vi "GPS Trail.vi"() -> ()   [LabVIEW 2009]
uses:
  <vilib>/Platform/TimedLoop/XDataNode/XDataNode.xnode
  <vilib>/Platform/TimedLoop/XDataNode/nitl_modes.ctl
  <vilib>/Platform/TimedLoop/XDataNode/XDNodeRunTimeDep.lvlib
  <vilib>/Platform/TimedLoop/XDataNode/wakeup.ctl
  <vilib>/Platform/TimedLoop/XDataNode/timing_clust.ctl
  <vilib>/Platform/TimedLoop/XDataNode/loadlvalarms.vi
  <vilib>/Analysis/NI_AALBase.lvlib
  TypeDefs/Sensor TypeDefs/GPS Data.ctl
  Functional Global Variables/Actions for FG's.ctl
panel:
  out "Latitude point sample":dbl format="%0.2f"
  out "Longitude point sample":dbl format="%0.2f"
  out "Latitude Array":dbl[](array[numeric]) format="%#_12g"
  out "Longitude Array":dbl[](array[numeric]) format="%#_12g"
  in  "Buffer Size (Seconds)":i32=10
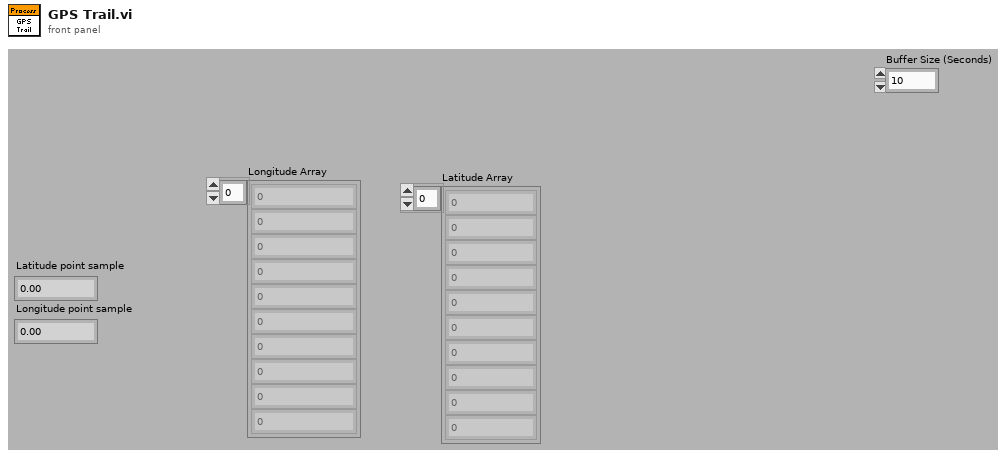
[diagram p1: front panel]
types:
  T1 = typedef "GPS Data.ctl" = cluster{"Latitude":dbl, "Longitude":dbl}
  T2 = typedef "XDNodeRunTimeDep.lvlib/timing_clust.ctl" = cluster{"Expected End [f-1]":u64, "Actual End [f-1]":u64, "Finished Late? [f-1]":bool, "Expected End [i-1]":u64, "Actual End [i-1]":u64, "Finished Late? [i-1]":bool, "Expected Start [i]":u64, "Actual Start [i]":u64, "Expected Start [f]":u64, "Actual Start [f]":u64, "Source Name":string, "Structure Name":string, "Period":i64, "Deadline":i64, "Offset":i64, "Start":i64, "Priority":i32, "Timeout":i32, "Mode":T3, "Wakeup Reason":T4, "Error":errorcluster, "Source Type":string, "Secondary Source Type":string, "Global End Time":u64, "Global Start Time":u64, "Frame Duration":u64, "Iteration Duration":u64, "Assigned CPU":i32, "I/O Scan Engine Mode":u32}
  T3 = typedef "XDNodeRunTimeDep.lvlib/nitl_modes.ctl" = enum32{"No Change", "Process missed periods, maintain original phase", "Discard missed periods, maintain original phase", "Process missed periods, ignore original phase", "Discard missed periods, ignore original phase"}
  T4 = typedef "XDNodeRunTimeDep.lvlib/wakeup.ctl" = enum32{"Normal", "Aborted", "Asynchronous wakeup", "Timing source error", "Timed loop error", "Timeout"}
  T5 = typedef "Actions for FG's.ctl" = enum16{"Read", "Write"}
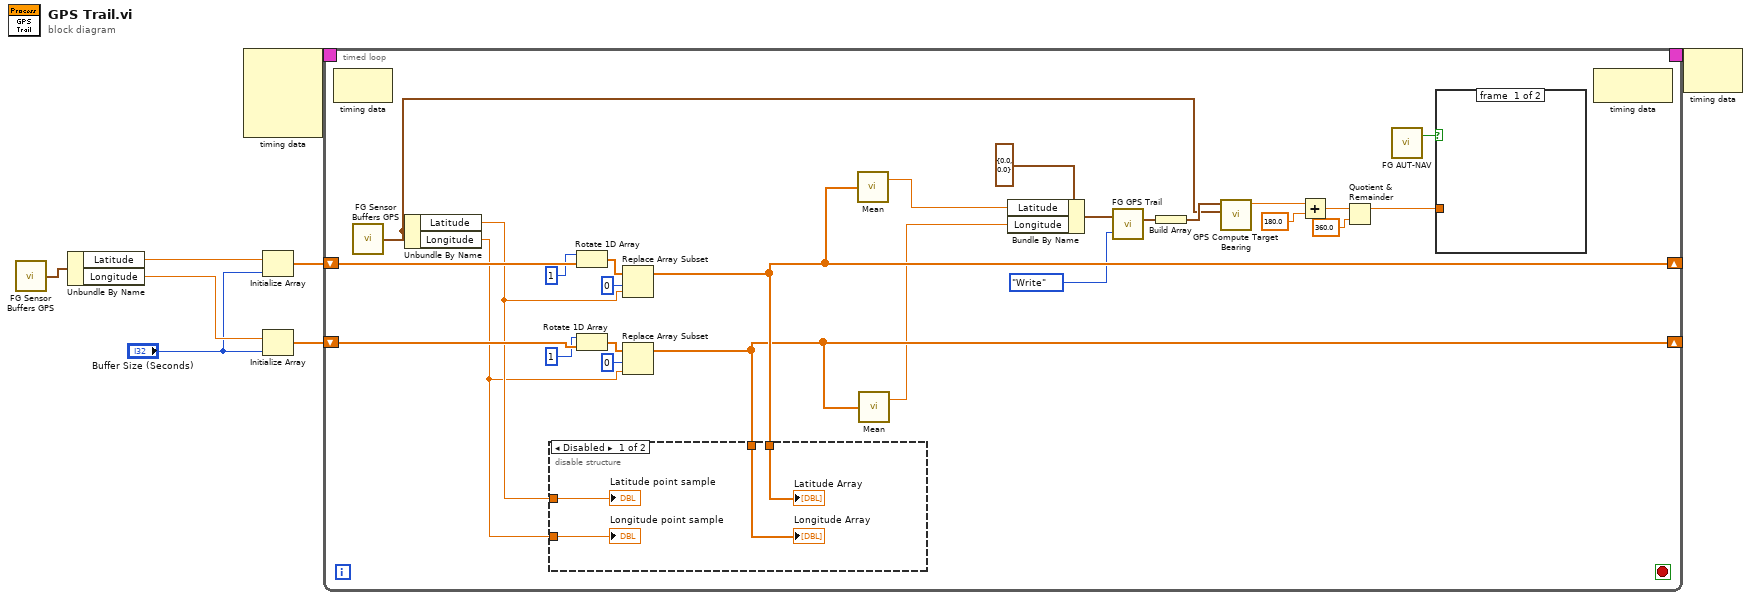
[diagram p0: block diagram]
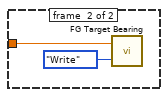
[diagram p3: hidden frame]
diagram:
  n1 = call "FG Sensor Buffers GPS.vi"() -> ("GPS Buffer out"=w6:T1)  [unwired: 2 in]
  n2 = Unbundle By Name(w6) -> ("Latitude"=w5:dbl, "Longitude"=w4:dbl)
  n3 = node-c288() -> (w8:T2)  [unwired: 4 in]
  n4 = Initialize Array(w5, "Buffer Size (Seconds)") -> (w3:dbl[])
  n5 = Initialize Array(w4, "Buffer Size (Seconds)") -> (w2:dbl[])
  n6 = timed-loop {
    timing: w8 -> [_]
    timing-out: [_] -> w7
    shift-right: [w24] -> _
    shift-left: w3 -> [w34]
    shift-right: [w23] -> _
    shift-left: w2 -> [w33]
    stop <- _ stop-if-true
    n7 = node-c288() -> ()  [unwired: 1 in, 1 out]
    n8 = call "FG Sensor Buffers GPS.vi"() -> ("GPS Buffer out"=w14:T1)  [unwired: 2 in]
    n9 = Unbundle By Name(w14) -> ("Latitude"=w32:dbl, "Longitude"=w31:dbl)
    n10 = Rotate 1D Array(1:w34, 2:1 ("n")) -> (0:w28:dbl[])
    n11 = Rotate 1D Array(1:w33, 2:1 ("n")) -> (0:w27:dbl[])
    n12 = Replace Array Subset(array=w28, new element=w32, index=0) -> (w24:dbl[])
    n13 = Replace Array Subset(array=w27, new element=w31, index=0) -> (w23:dbl[])
    n14 = disable-structure shown="Disabled" {
      disable-tunnel: w32 -> [w38 _]
      disable-tunnel: w31 -> [w37 _]
      disable-tunnel: w24 -> [w36 _]
      disable-tunnel: w23 -> [w35 _]
      frame #0 {
        "Latitude point sample" <- w38
        "Longitude point sample" <- w37
        "Latitude Array" <- w36
        "Longitude Array" <- w35
      }
      frame #1 {
      }
    }
    n15 = call <vilib>:"Mean.vi"("X"=w24) -> ("mean"=w21:dbl)  [unwired: 1 out]
    n16 = call <vilib>:"Mean.vi"("X"=w23) -> ("mean"=w20:dbl)  [unwired: 1 out]
    n17 = Bundle By Name(cluster=T1 {"Latitude"=0.0, "Longitude"=0.0} ("GPS Buffer out"), "Latitude"=w21, "Longitude"=w20) -> (w19:T1)
    n18 = call "FG GPS Trail.vi"("FG Action (Read)"=Actions_for_FG's."Write", "GPS Buffer in"=w19) -> ("GPS Buffer out"=w16:T1)  [unwired: 1 in]
    n19 = Build Array(w16) -> (w15:T1[])
    n20 = call "GPS Compute Target Bearing.vi"("Current co-ordinates"=w14, "GPS Waypoint List Out"=w15) -> ("Target Bearing (degrees)"=w13:dbl)  [unwired: 8 in]
    n21 = Add(x=w13, y=180.0) -> (x+y=w11:dbl)
    n22 = Quotient & Remainder(x=w11, y=360.0) -> (x-y*floor(x/y)=w10:dbl)  [unwired: 1 out]
    n23 = call "FG AUT-NAV.vi"() -> ("Aut/!Nav out"=w17:bool)  [unwired: 3 in]
    n24 = case shown="True" w17 {
      tunnel: w10 -> [_ w40]
      frame #0 {
      }
      frame #1 {
        n25 = call "FG Target Bearing.vi"("FG Action (Read)"=Actions_for_FG's."Write", "Target Bearing in"=w40) -> ()  [unwired: 1 out]
      }
    }
    n26 = node-c288() -> ()  [unwired: 1 in, 1 out]
  }
  n27 = node-c288(w7) -> ()  [unwired: 1 out]
